vi "Symphony Bin Axis.vi"(1 "Binning Factor":i32, 2 "Axis In":dbl[](array[numeric])) -> (0 "Axis Out":dbl[](array[numeric]))   [LabVIEW 2010]
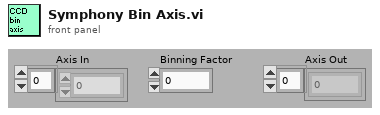
[diagram p1: front panel]
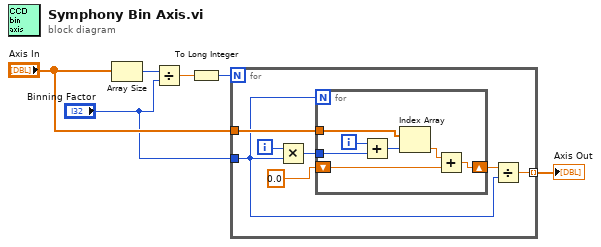
[diagram p0: block diagram]
diagram:
  n1 = Array Size(array="Axis In") -> (size(s)=w2:i32)
  n2 = Divide(x=w2, y="Binning Factor") -> (x/y=w1:dbl)
  n3 = To Long Integer(number=w1) -> (32bit integer=w3:i32)
  n4 = for {
    N: w3 -> [_]
    tunnel: "Binning Factor" -> [w9]
    tunnel: "Axis In" -> [w13]
    tunnel: [w10] -> w6 mode=indexing
    i -> [w8]
    n5 = Multiply(x=w8, y=w9) -> (x*y=w12:i32)
    n6 = for {
      N: w9 -> [_]
      tunnel: w13 -> [w20]
      tunnel: w12 -> [w17]
      shift-right: [w15] -> w11
      shift-left: 0.0 -> [w14]
      i -> [w18]
      n7 = Add(x=w18, y=w17) -> (x+y=w19:i32)
      n8 = Index Array(array=w20, index=w19) -> (element=w16:dbl)
      n9 = Add(x=w16, y=w14) -> (x+y=w15:dbl)
    }
    n10 = Divide(x=w11, y=w9) -> (x/y=w10:dbl)
  }
  "Axis Out" <- w6
